vi "Segment 0 Coder.vi"(9 "Segment 0":T1, 10 "File ID":string, 11 "仪器地址":u32) -> (3 "Output":string)   [LabVIEW 2010, in "DCP551.lvlib"]
uses:
  DCP551.lvlib
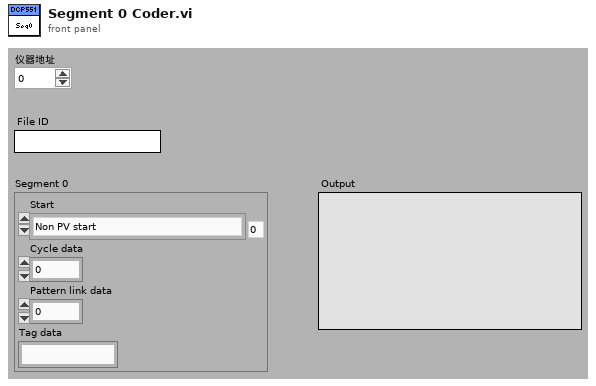
[diagram p1: front panel]
types:
  T1 = cluster{"Start":enum16{"Non PV start", "Upward PV tart", "Downward PV start", "Either upward of downward PV start"}, "Cycle data":i32, "Pattern link data":i32, "Tag data":string}
  T2 = enum16{"Non PV start", "Upward PV tart", "Downward PV start", "Either upward of downward PV start"}
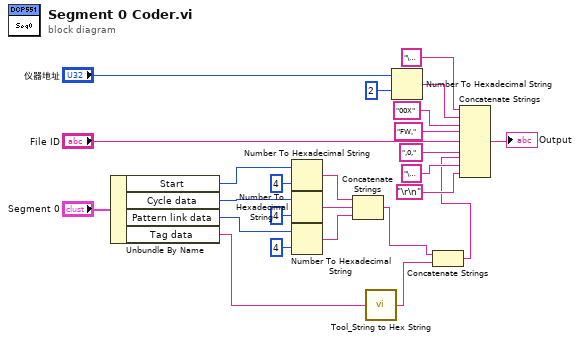
[diagram p0: block diagram]
diagram:
  n1 = Unbundle By Name("Segment 0") -> ("Start"=w21:T2, "Cycle data"=w20:i32, "Pattern link data"=w19:i32, "Tag data"=w1:string)
  n2 = Number To Hexadecimal String(1:i16 4 ("width (-)"), 2:w21) -> (0:w18:string)
  n3 = Number To Hexadecimal String(1:i16 4 ("width (-)"), 2:w20) -> (0:w17:string)
  n4 = Number To Hexadecimal String(1:i16 4 ("width (-)"), 2:w19) -> (0:w16:string)
  n5 = Concatenate Strings(w18, w17, w16) -> (w4:string)
  n6 = call "Tool_String to Hex String.vi"("String"=w1) -> ("Hex String"=w2:string)  [unwired: 14 in]
  n7 = Number To Hexadecimal String(1:i16 2 ("width (-)"), 2:"仪器地址") -> (0:w8:string)
  n8 = Concatenate Strings(w4, w2) -> (w3:string)
  n9 = Concatenate Strings("\u0002" ("string"), w8, "00X" ("string"), "FW," ("string"), "File ID", ",0," ("string"), w3, "\u0003" ("string"), "\r\n") -> (→"Output":string)
